vi "Teleop.vi"(10 "Match Info":T3={"Autonomous Elapsed Seconds"=0.0, "TeleOp Elapsed Seconds"=0.0, "Disabled Elapsed Seconds"=0.0, "Visited Autonomous"=FALSE, "Visited TeleOp"=FALSE, "Visited Disabled"=FALSE, "Autonomous Settings"={"Autonomous Style"=enum."Independent", "VI Refnum"=refnum}}, 11 "Call Context":T4) -> ()   [LabVIEW 2020]
doc: "This VI is called for each TeleOp packet received from the DS where the robot is not disabled. It is often used to read from the joysticks and update I/O or to update setpoints for timed control loops. It should complete and return within 20 milliseconds or it may miss DS packets."
uses:
  <vilib>/Rock Robotics/WPI/DriverStation/WPI_DriverStationDerivedRobotMode.ctl
  <vilib>/Rock Robotics/WPI/DriverStation/WPI_DriverStationMatch Info.ctl
  <vilib>/Rock Robotics/WPI/Solenoid/WPI_SolenoidValue.ctl
  <vilib>/Rock Robotics/WPI/ThirdParty/Phoenix-LabVIEW/Motor Controller/Controls/CTRE_Phoenix_MotorControl_ControlMode.ctl
  <vilib>/Rock Robotics/WPI/Utilities/WPI_GetSetVariantRefNum.vi
  <vilib>/Rock Robotics/WPI/ThirdParty/Phoenix-LabVIEW/Pigeon IMU/CTRE_PigeonIMU_GetYPR.vi
  <vilib>/Rock Robotics/Network Tables/NT Read Boolean.vi
  <vilib>/Rock Robotics/Network Tables/NT Read Number.vi
  <vilib>/Rock Robotics/Network Tables/NT Write String.vi
  <vilib>/Rock Robotics/Network Tables/NT Read String.vi
  <vilib>/Rock Robotics/Network Tables/NT Write Boolean.vi
  <vilib>/Rock Robotics/WPI/Solenoid/WPI_SolenoidSetEnum.vi
  <vilib>/Rock Robotics/WPI/ThirdParty/Phoenix-LabVIEW/Motor Controller/Get/CTRE_Phoenix_MotorController_IntegratedSensorData_TalonFX.vi
  <vilib>/Rock Robotics/WPI/ThirdParty/Phoenix-LabVIEW/CANCoder/Get/CTRE_Phoenix_CANcoder_GetSensorData.vi
  <vilib>/addons/control/pid/pid.llb/PID (DBL).vi
  <vilib>/addons/control/pid/NI_PID_pid.lvlib
panel:
  in  "ballCount":dbl
  out "Pigeon Value":dbl
  out "frontrightmotor":dbl
  out "frontleftdrive":dbl
  in  "PID gains 4":T1={"proportional gain (Kc)"=-0.01, "integral time (Ti, min)"=0.0, "derivative time (Td, min)"=2e-05} {"derivative time (Td, min)" format="%.6f"; "integral time (Ti, min)" format="%.6f"; "proportional gain (Kc)" format="%.6f"}
  in  "PID gains 3":T1={"proportional gain (Kc)"=0.01, "integral time (Ti, min)"=0.0, "derivative time (Td, min)"=2e-05} {"derivative time (Td, min)" format="%.6f"; "integral time (Ti, min)" format="%.6f"; "proportional gain (Kc)" format="%.6f"}
  in  "PID gains 2":T1={"proportional gain (Kc)"=-0.01, "integral time (Ti, min)"=0.0, "derivative time (Td, min)"=2e-05} {"derivative time (Td, min)" format="%.6f"; "integral time (Ti, min)" format="%.6f"; "proportional gain (Kc)" format="%.6f"}
  in  "PID gains":T1={"proportional gain (Kc)"=0.01, "integral time (Ti, min)"=0.0, "derivative time (Td, min)"=2e-05} {"derivative time (Td, min)" format="%.6f"; "integral time (Ti, min)" format="%.6f"; "proportional gain (Kc)" format="%.6f"}
  out "Motor out 4":dbl
  out "Desired Position 4":dbl
  out "Motor out 1":dbl
  out "Desired Position 1":dbl
  out "Motor Out 2":dbl
  out "Desired Position 2":dbl
  out "Motor out 3":dbl
  out "Desired Position 3":dbl
  out "Sensor Position 4":dbl
  out "Sensor Position 3":dbl
  out "Sensor Position 2":dbl
  out "Sensor Position 1":dbl
  out "Rotation steering angle 4":dbl
  out "WheelDirection4":dbl(knob) scale=180.0..-180.0
  out "Throttle 4":dbl(slide) scale=-1.0..1.0
  out "Y4":dbl
  out "X4":dbl
  out "Rotation steering angle 3":dbl
  out "WheelDirection3":dbl(knob) scale=180.0..-180.0
  out "Throttle 3":dbl(slide) scale=-1.0..1.0
  out "Y3":dbl
  out "X3":dbl
  out "Rotation steering angle 2":dbl
  out "WheelDirection2":dbl(knob) scale=180.0..-180.0
  out "Throttle 2":dbl(slide) scale=-1.0..1.0
  out "Y2":dbl
  out "X2":dbl
  out "Rotation steering angle 1":dbl
  out "WheelDirection1":dbl(knob) scale=180.0..-180.0
  out "Throttle 1":dbl(slide) scale=-1.0..1.0
  out "Y1":dbl
  out "X1":dbl
  out "Z - Axis":dbl
  out "Y - Axis":dbl
  out "X - Axis":dbl
  in  "Turret 2":dbl format="%#_13g"
  in  "Turret 1":dbl
  in  "Shoot %":dbl
  out "Limit 2":bool
  out "Limit 1":bool
  in  "intake press":T2=enum."Forward"
  in  "intake not press":T2=enum."Reverse"
  out "Position":dbl format="%.2f"
  in  "Elevate Wanted":dbl
  out "Elevate Pressed":bool
  out "Reject Pressed Count":i32
  in  "Elevate (not wanted)":dbl format="%#_13g"
  in  "Intake (wanted)":dbl=1.0 format="%#_13g"
  in  "Reject (wanted)":dbl=-1.0 format="%#_13g"
  in  "Reject (not wanted)":dbl
  in  "Intake (not wanted)":dbl
  in  "Auto-Accept":bool
  in  "8togglePressed?":bool
  in  "Red/Blue":u32(colorbox)
  out "B":u8
  out "G":u8
  out "R":u8
  out "Color":u32(colorbox)
  out "Sample Slider 0":dbl(slide) scale=0.0..5.0
  out "Sample Boolean 1":bool
  out "Sample Boolean 0":bool
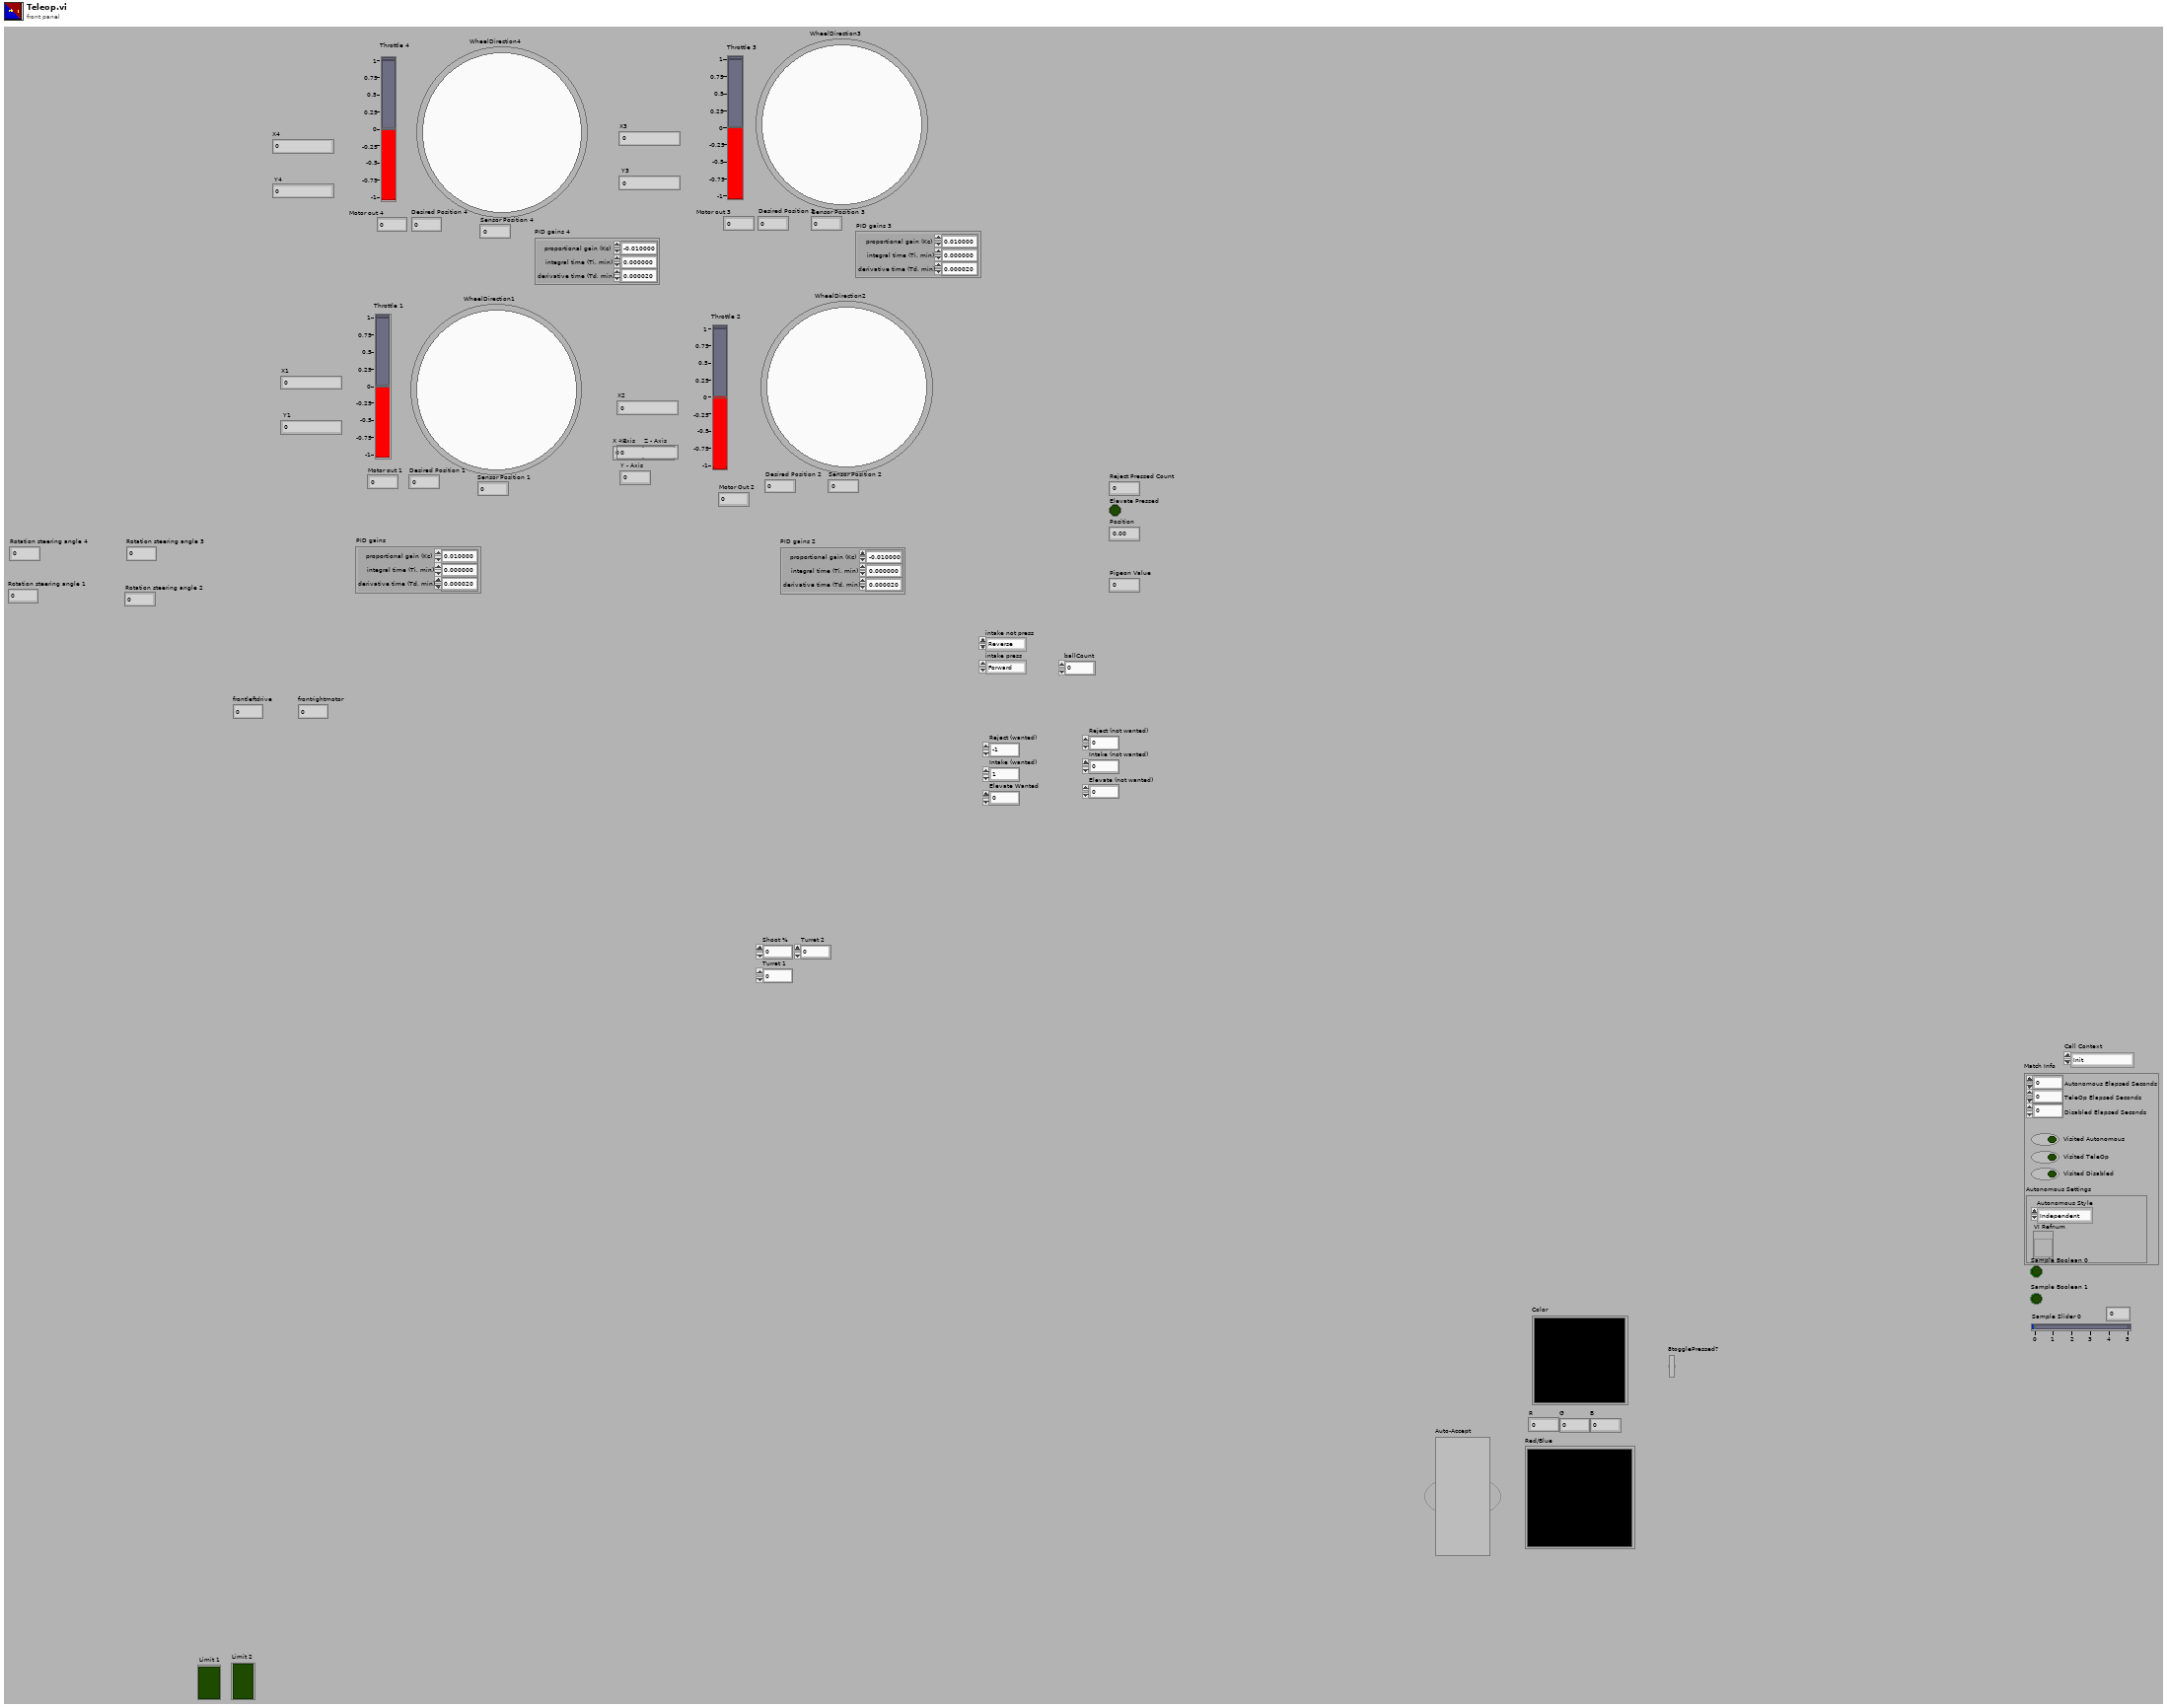
[diagram p1: front panel]
types:
  T1 = cluster{"proportional gain (Kc)":dbl, "integral time (Ti, min)":dbl, "derivative time (Td, min)":dbl}
  T2 = typedef "WPI_SolenoidValue.ctl" = enum16{"Off", "On", "Forward", "Reverse"}
  T3 = typedef "WPI_DriverStationMatch Info.ctl" = cluster{"Autonomous Elapsed Seconds":dbl, "TeleOp Elapsed Seconds":dbl, "Disabled Elapsed Seconds":dbl, "Visited Autonomous":bool, "Visited TeleOp":bool, "Visited Disabled":bool, "Autonomous Settings":cluster{"Autonomous Style":enum16{"Iterative", "Independent"}, "VI Refnum":refnum<vi>}}
  T4 = typedef "WPI_DriverStationDerivedRobotMode.ctl" = enum16{"Init", "Execute", "Stop"}
  T5 = typedef "CTRE_Phoenix_MotorControl_ControlMode.ctl" = u16
  T6 = typedef "WPI_MotorControlDeviceRef.ctl" = cluster{"DeviceStatus":errorcluster, "Type":T7, "PWM":cluster{"PWM Channel":T8, "DeadBand":T9}, "CAN":cluster{"Device Number":u8, "SetOutput VI Ref":variant, "GetOutput VI Ref":variant, "Enable VI Ref":variant, "Disable VI Ref":variant, "Data":variant}, "Invert":bool, "DIO PWM":cluster{"PWM \"Enable\" Channel":T8, "DIOChannel":T10, "PWM Rate":dbl}}
  T7 = typedef "WPI_MotorControlType.ctl" = enum16{"PWM", "CAN", "DIO PWM"}
  T8 = typedef "FPGA_DIOPWMChannel.ctl" = enum8{"PWM 0", "PWM 1", "PWM 2", "PWM 3", "PWM 4", "PWM 5", "PWM 6", "PWM 7", "PWM 8", "PWM 9", "PWM MXP 0", "PWM MXP 1", "PWM MXP 2", "PWM MXP 3", "PWM MXP 4", "PWM MXP 5", "PWM MXP 6", "PWM MXP 7", "PWM MXP 8", "PWM MXP 9", "Invalid"}
  T9 = typedef "WPI_PWMDeadband.ctl" = cluster{"Name":string, "maxPositivePwm":i32, "minPositivePwm":i32, "centerPwm":i32, "maxNegativePwm":i32, "minNegativePwm":i32, "angularRange":u16}
  T10 = typedef "FPGA_DIOChannel.ctl" = enum8{"DIO 0", "DIO 1", "DIO 2", "DIO 3", "DIO 4", "DIO 5", "DIO 6", "DIO 7", "DIO 8", "DIO 9", "DIO MXP 0", "DIO MXP 1", "DIO MXP 2", "DIO MXP 3", "DIO MXP 4", "DIO MXP 5", "DIO MXP 6", "DIO MXP 7", "DIO MXP 8", "DIO MXP 9", "DIO MXP 10", "DIO MXP 11", "DIO MXP 12", "DIO MXP 13", "DIO MXP 14", "DIO MXP 15", "SPI Port CS1", "SPI Port CS2", "SPI Port CS3", "SPI Port MISO", "SPI Port MOSI", "Invalid"}
  T11 = typedef "WPI_SwitchDevRef.ctl" = cluster{"DevStatus":errorcluster, "DIO Channel":T10, "CntIndex":T12, "Normally Closed":bool}
  T12 = typedef "FPGA_CounterCtrSystemIndex.ctl" = enum8{"Ctr 0", "Ctr 1", "Ctr 2", "Ctr 3", "Ctr 4", "Ctr 5", "Ctr 6", "Ctr 7", "Invalid"}
  T13 = typedef "WPI_SolenoidDevRef.ctl" = cluster{"DevStatus":errorcluster, "Pneumatics Control Module":u8, "Forward Solenoid Channel":T14, "Reverse Solenoid Channel":T14}
  T14 = typedef "WPI_SolenoidChannel.ctl" = enum8{"Solenoid 0", "Solenoid 1", "Solenoid 2", "Solenoid 3", "Solenoid 4", "Solenoid 5", "Solenoid 6", "Solenoid 7", "Solenoid 8", "Solenoid 9", "Solenoid 10", "Solenoid 11", "Solenoid 12", "Solenoid 13", "Solenoid 14", "Solenoid 15", "Invalid"}
  T15 = typedef "Color Sensor V3 DevRef.ctl" = cluster{"I2CDevRef":T16}
  T16 = typedef "WPI_I2CDevRef.ctl" = cluster{"DevStatus":errorcluster, "Device Address":u8, "Handle":i32, "I2C Bus":T17}
  T17 = typedef "i2c_bus.ctl" = enum16{"I2C On-Board", "I2C MXP", "Invalid"}
  T18 = typedef "WPI_JoystickDevRef.ctl" = cluster{"Device":T19}
  T19 = typedef "WPI_JoystickDeviceEnum.ctl" = enum16{"USB 0", "USB 1", "USB 2", "USB 3", "USB 4", "USB 5"}
  T20 = typedef "CTRE_PigeonIMU_DeviceRef.ctl" = cluster{"DeviceStatus":errorcluster, "Device Number":u8, "Type":T21, "Device ID":u32, "Handle":u64, "UsageFrame":u32, "Library Path":path}
  T21 = typedef "CTRE_PigeonIMU_ConnectionType.ctl" = u32
  T22 = typedef "WPI_CompressorDevRef.ctl" = cluster{"DevStatus":errorcluster, "Pneumatics Control Module":u8}
  T23 = typedef "CTRE_Phoenix_CANcoder_DeviceRef.ctl" = cluster{"DeviceStatus":errorcluster, "Device Number":u8, "Handle":u64, "UsageFrame":u32, "Library Path":path}
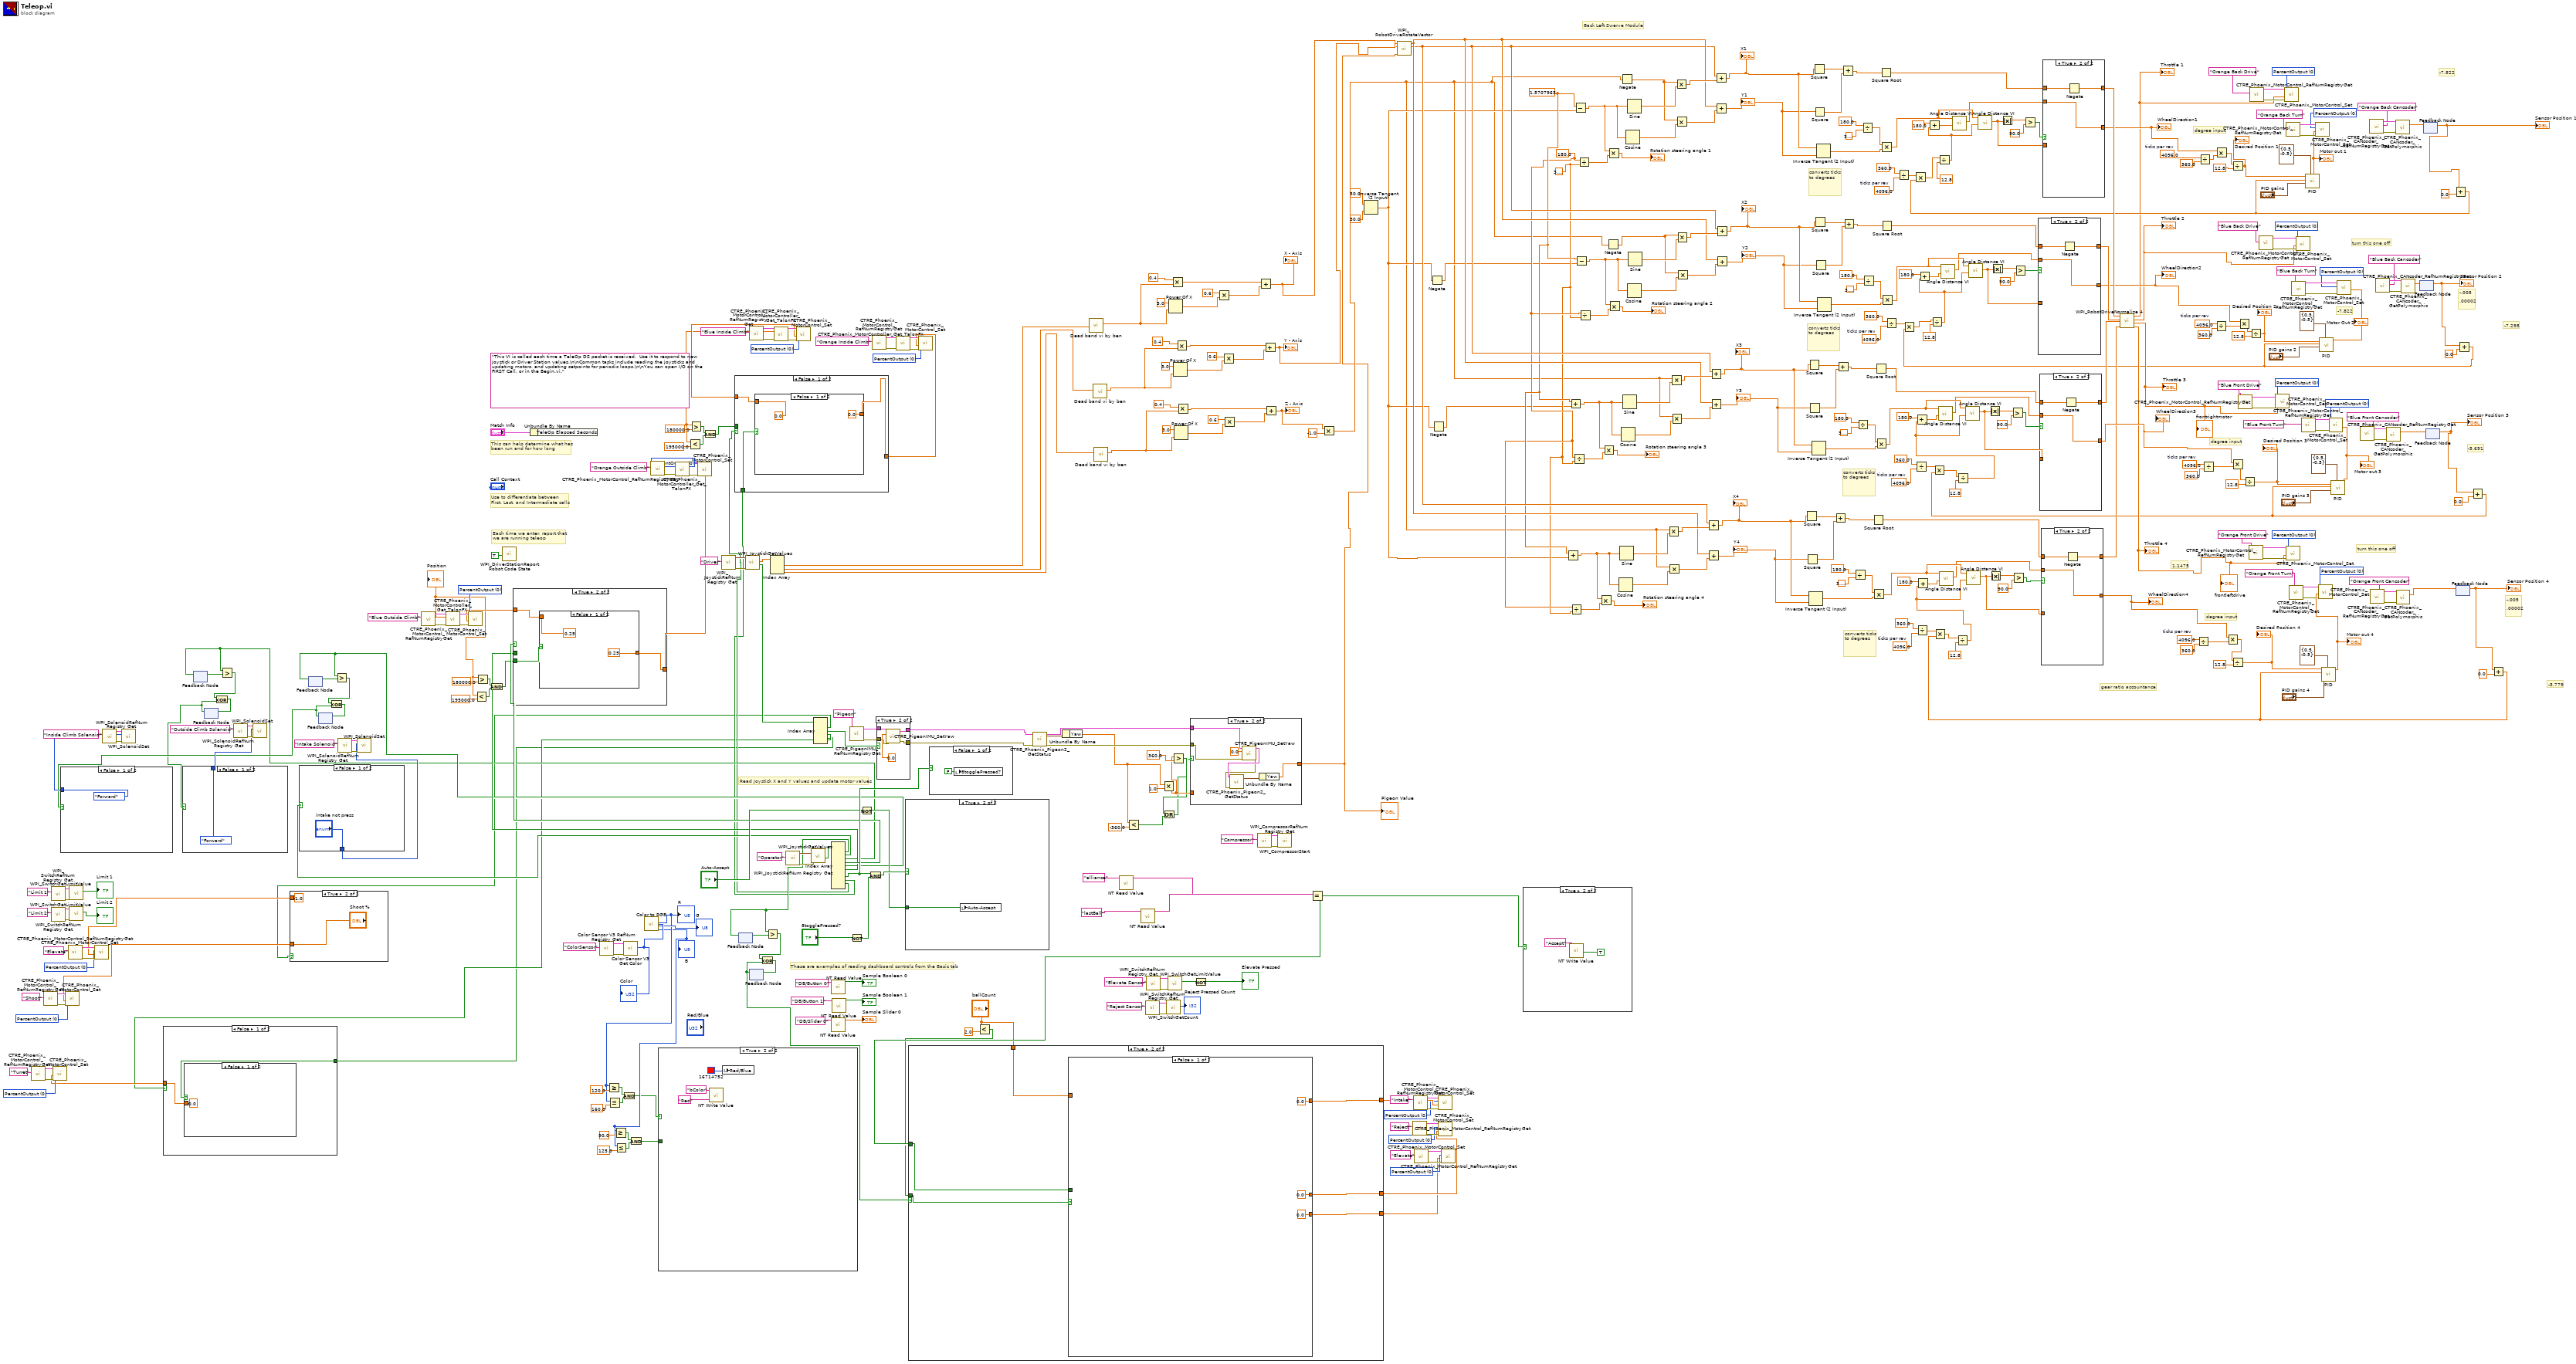
[diagram p0: block diagram]
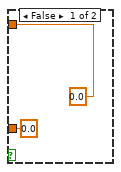
[diagram p2: hidden frame]
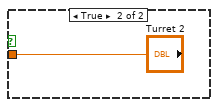
[diagram p8: hidden frame]
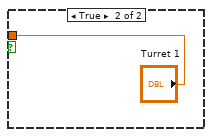
[diagram p9: hidden frame]
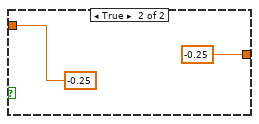
[diagram p10: hidden frame]
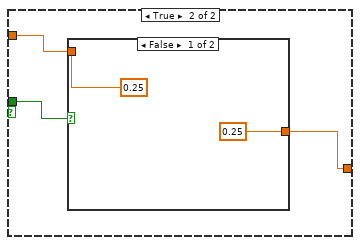
[diagram p11: hidden frame]
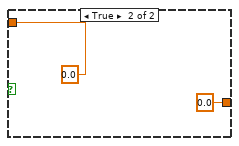
[diagram p12: hidden frame]
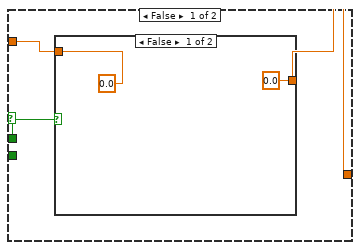
[diagram p13: hidden frame]
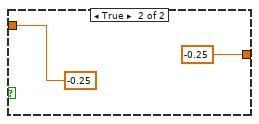
[diagram p14: hidden frame]
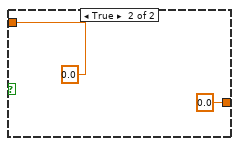
[diagram p15: hidden frame]
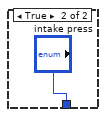
[diagram p16: hidden frame]
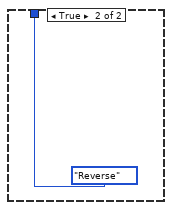
[diagram p17: hidden frame]
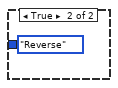
[diagram p18: hidden frame]
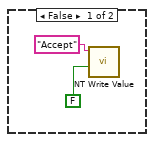
[diagram p19: hidden frame]
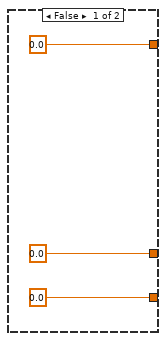
[diagram p20: hidden frame]
diagram:
  w20 = T5 0 items=["PercentOutput"=0, "Position"=1, "Velocity"=2, "Current"=3, "Follower"=5, "MotionProfile"=6, "MotionMagic"=7, "MotionProfileArc"=10, "Disabled"=15] ("Control Mode")
  w102 = T5 0 items=["PercentOutput"=0, "Position"=1, "Velocity"=2, "Current"=3, "Follower"=5, "MotionProfile"=6, "MotionMagic"=7, "MotionProfileArc"=10, "Disabled"=15] ("Control Mode")
  w114 = T5 0 items=["PercentOutput"=0, "Position"=1, "Velocity"=2, "Current"=3, "Follower"=5, "MotionProfile"=6, "MotionMagic"=7, "MotionProfileArc"=10, "Disabled"=15] ("Control Mode")
  w115 = T5 0 items=["PercentOutput"=0, "Position"=1, "Velocity"=2, "Current"=3, "Follower"=5, "MotionProfile"=6, "MotionMagic"=7, "MotionProfileArc"=10, "Disabled"=15] ("Control Mode")
  w116 = T5 0 items=["PercentOutput"=0, "Position"=1, "Velocity"=2, "Current"=3, "Follower"=5, "MotionProfile"=6, "MotionMagic"=7, "MotionProfileArc"=10, "Disabled"=15] ("Control Mode")
  w117 = T5 0 items=["PercentOutput"=0, "Position"=1, "Velocity"=2, "Current"=3, "Follower"=5, "MotionProfile"=6, "MotionMagic"=7, "MotionProfileArc"=10, "Disabled"=15] ("Control Mode")
  w118 = T5 0 items=["PercentOutput"=0, "Position"=1, "Velocity"=2, "Current"=3, "Follower"=5, "MotionProfile"=6, "MotionMagic"=7, "MotionProfileArc"=10, "Disabled"=15] ("Control Mode")
  w119 = T5 0 items=["PercentOutput"=0, "Position"=1, "Velocity"=2, "Current"=3, "Follower"=5, "MotionProfile"=6, "MotionMagic"=7, "MotionProfileArc"=10, "Disabled"=15] ("Control Mode")
  w120 = T5 0 items=["PercentOutput"=0, "Position"=1, "Velocity"=2, "Current"=3, "Follower"=5, "MotionProfile"=6, "MotionMagic"=7, "MotionProfileArc"=10, "Disabled"=15] ("Control Mode")
  w132 = 4096.0  # ticks per rev
  w145 = 4096.0  # ticks per rev
  w159 = 4096.0  # ticks per rev
  w170 = 4096.0  # ticks per rev
  w62 = 1.5707963 ("y")
  w181 = 4096.0  # ticks per rev
  w185 = 4096.0  # ticks per rev
  w189 = 4096.0  # ticks per rev
  w105 = 4096.0  # ticks per rev
  w60 = 3.141592653589793
  w61 = 180.0 ("x")
  w299 = T5 0 items=["PercentOutput"=0, "Position"=1, "Velocity"=2, "Current"=3, "Follower"=5, "MotionProfile"=6, "MotionMagic"=7, "MotionProfileArc"=10, "Disabled"=15] ("Control Mode")
  w303 = T5 0 items=["PercentOutput"=0, "Position"=1, "Velocity"=2, "Current"=3, "Follower"=5, "MotionProfile"=6, "MotionMagic"=7, "MotionProfileArc"=10, "Disabled"=15] ("Control Mode")
  w327 = T5 0 items=["PercentOutput"=0, "Position"=1, "Velocity"=2, "Current"=3, "Follower"=5, "MotionProfile"=6, "MotionMagic"=7, "MotionProfileArc"=10, "Disabled"=15] ("Control Mode")
  w328 = T5 0 items=["PercentOutput"=0, "Position"=1, "Velocity"=2, "Current"=3, "Follower"=5, "MotionProfile"=6, "MotionMagic"=7, "MotionProfileArc"=10, "Disabled"=15] ("Control Mode")
  w329 = T5 0 items=["PercentOutput"=0, "Position"=1, "Velocity"=2, "Current"=3, "Follower"=5, "MotionProfile"=6, "MotionMagic"=7, "MotionProfileArc"=10, "Disabled"=15] ("Control Mode")
  w369 = T5 0 items=["PercentOutput"=0, "Position"=1, "Velocity"=2, "Current"=3, "Follower"=5, "MotionProfile"=6, "MotionMagic"=7, "MotionProfileArc"=10, "Disabled"=15] ("Control Mode")
  w402 = T5 0 items=["PercentOutput"=0, "Position"=1, "Velocity"=2, "Current"=3, "Follower"=5, "MotionProfile"=6, "MotionMagic"=7, "MotionProfileArc"=10, "Disabled"=15] ("Control Mode")
  w403 = T5 0 items=["PercentOutput"=0, "Position"=1, "Velocity"=2, "Current"=3, "Follower"=5, "MotionProfile"=6, "MotionMagic"=7, "MotionProfileArc"=10, "Disabled"=15] ("Control Mode")
  w407 = T5 0 items=["PercentOutput"=0, "Position"=1, "Velocity"=2, "Current"=3, "Follower"=5, "MotionProfile"=6, "MotionMagic"=7, "MotionProfileArc"=10, "Disabled"=15] ("Control Mode")
  (unwired) "This VI is called each time a TeleOp DS packet is received.  Use it to respond to new joystick or Driver Station values.\n\nCommon tasks include reading the joysticks and updating motors, and updating setpoints for periodic loops.\n\nYou can open I/O on the FIRST Call, or in the Begin.vi."
  # "-.005\n\n.00002"
  # "-.005\n\n.00002"
  # "-7.822"
  # "-7.295"
  # "-3.691"
  # "-3.779"
  # "1.1475"
  # "turn this one off"
  # "turn this one off"
  # "gear ratio accountance"
  # "converts ticks to degrees"
  # "converts ticks to degrees"
  # "converts ticks to degrees"
  # "converts ticks to degrees"
  # "degree input"
  # "degree input"
  # "degree input"
  # "Back Left Swerve Module"
  # "These are examples of reading dashboard controls from the Basic tab"
  # "Read Joystick X and Y values and update motor values"
  # "-7.822"
  # "Each time we enter, report that\nwe are running teleop"
  # "Use to differentiate between\nFirst, Last, and Intermediate calls"
  # "This can help determine what has\nbeen run and for how long"
  n1 = call <vilib>:"CTRE_Phoenix_MotorControl_RefNumRegistryGet.vi"("refnum name"="Turret") -> ("error out"=w302:errorcluster, "PhoenixMotorControlDevRef"=w301:T6)  [unwired: 9 in]
  n2 = call <vilib>:"CTRE_Phoenix_MotorControl_RefNumRegistryGet.vi"("refnum name"="Shoot") -> ("error out"=w306:errorcluster, "PhoenixMotorControlDevRef"=w305:T6)  [unwired: 9 in]
  n3 = call <vilib>:"WPI_SwitchRefNum Registry Get.vi"("refnum name"="Limit 1") -> ("error out"=w314:errorcluster, "SwitchDevRef"=w313:T11)  [unwired: 9 in]
  n4 = call <vilib>:"WPI_SwitchRefNum Registry Get.vi"("refnum name"="Limit 2") -> ("error out"=w311:errorcluster, "SwitchDevRef"=w310:T11)  [unwired: 9 in]
  n5 = call <vilib>:"CTRE_Phoenix_MotorControl_RefNumRegistryGet.vi"("refnum name"="Elevate") -> ("error out"=w22:errorcluster, "PhoenixMotorControlDevRef"=w19:T6)  [unwired: 9 in]
  n6 = call <vilib>:"WPI_SwitchGetLimitValue.vi"("error in (no error)"=w314, "SwitchDevRef"=w313) -> ("Switch Pressed"=→"Limit 1":bool)  [unwired: 7 in, 2 out]
  n7 = call <vilib>:"WPI_SwitchGetLimitValue.vi"("error in (no error)"=w311, "SwitchDevRef"=w310) -> ("Switch Pressed"=→"Limit 2":bool)  [unwired: 7 in, 2 out]
  n8 = call <vilib>:"WPI_SolenoidRefNum Registry Get.vi"("refnum name"="Inside Climb Solenoid") -> ("error out"=w386:errorcluster, "SolenoidDevRef"=w385:T13)  [unwired: 9 in]
  n9 = feedback #1() -> (w349:bool)  [unwired: 1 in]
  n10 = feedback #2() -> (w345:bool)  [unwired: 1 in]
  n11 = case shown="False" w345 {
    tunnel: [WPI_SolenoidValue."Forward" ("Value") WPI_SolenoidValue."Reverse" ("Value")] -> w376
    frame False {
    }
    frame True {
    }
  }
  n12 = call <vilib>:"WPI_SolenoidRefNum Registry Get.vi"("refnum name"="Outside Climb Solenoid") -> ("error out"=w384:errorcluster, "SolenoidDevRef"=w383:T13)  [unwired: 9 in]
  n13 = call-poly <vilib>:"WPI_SolenoidSet.vi"("error in (no error)"=w384, "Value"=w376, "SolenoidDevRef"=w383) -> ()  [unwired: 7 in, 2 out]
  n14 = feedback #3() -> (w354:bool)  [unwired: 1 in]
  n15 = feedback #4() -> (w350:bool)  [unwired: 1 in]
  n16 = case shown="False" w350 {
    tunnel: [WPI_SolenoidValue."Forward" ("Value") WPI_SolenoidValue."Reverse" ("Value")] -> w377
    frame False {
    }
    frame True {
    }
  }
  n17 = call-poly <vilib>:"WPI_SolenoidSet.vi"("error in (no error)"=w386, "Value"=w377, "SolenoidDevRef"=w385) -> ()  [unwired: 7 in, 2 out]
  n18 = call <vilib>:"WPI_SolenoidRefNum Registry Get.vi"("refnum name"="Intake Solenoid") -> ("error out"=w382:errorcluster, "SolenoidDevRef"=w381:T13)  [unwired: 9 in]
  n19 = call <vilib>:"CTRE_Phoenix_MotorControl_RefNumRegistryGet.vi"("refnum name"="Blue Outside Climb") -> ("error out"=w372:errorcluster, "PhoenixMotorControlDevRef"=w373:T6)  [unwired: 9 in]
  n20 = call-poly <vilib>:"CTRE_Phoenix_MotorController_Get_TalonFX.vi"("PhoenixMotorControlDevRef"=w373, "error in"=w372) -> ("PhoenixMotorControlDevRef"=w370:T6, "Position"=w362:dbl, "error out"=w371:errorcluster)  [unwired: 9 in, 2 out]
  "Position" <- w362
  n21 = Less?(x=w362, y=195000.0) -> (x < y?=w363:bool)
  n22 = Greater?(x=w362, y=180000.0) -> (0:w364:bool)
  n23 = And(x=w364, y=w363) -> (x .and. y?=w317:bool)
  n24 = call <vilib>:"WPI_DriverStationReport Robot Code State.vi"("TeleOp"=TRUE ("Autonomous")) -> ()  [unwired: 10 in, 1 out]
  n25 = Unbundle By Name("Match Info") -> ()  [unwired: 1 out]
  n26 = call <vilib>:"Color Sensor V3 RefNum Registry Get.vi"("refnum name"="ColorSensor") -> ("error out"=w441:errorcluster, "ColorSensorDevRef"=w442:T15)  [unwired: 9 in]
  n27 = call <vilib>:"Color Sensor V3 Get Color.vi"("error in (no error)"=w441, "ColorSensorDevRef"=w442) -> ("Color"=w440:u32)  [unwired: 6 in, 3 out]
  "Color" <- w440
  n28 = call <vilib>:"Color to RGB.vi"("Color"=w440) -> ("R"=w434:u8, "G"=→"G":u8, "B"=w429:u8)  [unwired: 1 out]
  "R" <- w434
  "B" <- w429
  n29 = Greater Or Equal?(x=w434, y=120.0) -> (x >= y?=w437:bool)
  n30 = Less Or Equal?(x=w434, y=160.0) -> (x <= y?=w438:bool)
  n31 = Greater Or Equal?(x=w429, y=90.0) -> (x >= y?=w432:bool)
  n32 = Less Or Equal?(x=w429, y=125.0) -> (x <= y?=w433:bool)
  n33 = And(x=w437, y=w438) -> (x .and. y?=w418:bool)
  n34 = And(x=w432, y=w433) -> (x .and. y?=w417:bool)
  n35 = call <vilib>:"CTRE_Phoenix_MotorControl_RefNumRegistryGet.vi"("refnum name"="Orange Outside Climb") -> ("error out"=w333:errorcluster, "PhoenixMotorControlDevRef"=w334:T6)  [unwired: 9 in]
  n36 = case shown="True" w418 {
    tunnel: w417 -> [w469 _]
    frame False {
      n37 = case shown="True" w469 {
        frame False {
          n38 = call-poly <vilib>:"NT Write Value.vi"("String"="Empty", "Name"="bColor") -> ()  [unwired: 9 in, 1 out]
          n39 = local write "Red/Blue"(u32 328965 ("Color Box")) -> ()
        }
        frame True {
          n40 = local write "Red/Blue"(u32 1507583 ("Color Box")) -> ()
          n41 = call-poly <vilib>:"NT Write Value.vi"("String"="Blue", "Name"="bColor") -> ()  [unwired: 9 in, 1 out]
        }
      }
    }
    frame True {
      n42 = call-poly <vilib>:"NT Write Value.vi"("String"="Red", "Name"="bColor") -> ()  [unwired: 9 in, 1 out]
      n43 = local write "Red/Blue"(u32 16714752) -> ()
    }
  }
  n44 = call-poly <vilib>:"CTRE_Phoenix_MotorController_Get_TalonFX.vi"("PhoenixMotorControlDevRef"=w334, "error in"=w333) -> ("PhoenixMotorControlDevRef"=w331:T6, "error out"=w332:errorcluster)  [unwired: 9 in, 3 out]
  n45 = call <vilib>:"WPI_JoystickRefNum Registry Get.vi"("refnum name"="Driver") -> ("error out"=w462:errorcluster, "JoystickDevRef"=w461:T18)  [unwired: 9 in]
  n46 = feedback #5() -> (w359:bool)  [unwired: 1 in]
  n47 = call <vilib>:"WPI_JoystickGetValues.vi"("error in (no error)"=w462, "JoystickDevRef"=w461) -> ("Buttons"=w458:bool[], "Axes"=w459:dbl[])  [unwired: 5 in, 3 out]
  n48 = call <vilib>:"CTRE_Phoenix_MotorControl_RefNumRegistryGet.vi"("refnum name"="Blue Inside Climb") -> ("error out"=w338:errorcluster, "PhoenixMotorControlDevRef"=w339:T6)  [unwired: 9 in]
  n49 = feedback #6() -> (w355:bool)  [unwired: 1 in]
  n50 = Index Array(array=w459) -> (element #1=w25:dbl, element #2=w24:dbl, element #3=w23:dbl)  [unwired: 3 in]
  n51 = call-poly <vilib>:"CTRE_Phoenix_MotorController_Get_TalonFX.vi"("PhoenixMotorControlDevRef"=w339, "error in"=w338) -> ("PhoenixMotorControlDevRef"=w336:T6, "Position"=w318:dbl, "error out"=w337:errorcluster)  [unwired: 9 in, 2 out]
  n52 = Less?(x=w318, y=195000.0) -> (x < y?=w321:bool)
  n53 = Greater?(x=w318, y=180000.0) -> (0:w322:bool)
  n54 = And(x=w322, y=w321) -> (x .and. y?=w316:bool)
  n55 = call <vilib>:"WPI_JoystickRefNum Registry Get.vi"("refnum name"="Operator") -> ("error out"=w427:errorcluster, "JoystickDevRef"=w426:T18)  [unwired: 9 in]
  n56 = call <vilib>:"WPI_JoystickGetValues.vi"("error in (no error)"=w427, "JoystickDevRef"=w426) -> ("Buttons"=w425:bool[])  [unwired: 5 in, 4 out]
  n57 = Index Array(array=w458) -> (element #1=w4:bool, element #2=w455:bool, element #3=w297:bool, element #4=w296:bool)  [unwired: 5 in, 1 out]
  n58 = case shown="False" w297 {
    tunnel: [w480 "Turret 1"] -> w298
    tunnel: w296 -> [w479 _]
    frame False {
      n59 = case shown="False" w479 {
        tunnel: [0.0 ("Turret 2") "Turret 2"] -> w480
        frame False {
        }
        frame True {
        }
      }
    }
    frame True {
    }
  }
  n60 = call <vilib>:"CTRE_Phoenix_MotorControl_Set.vi"("error in (no error)"=w302, "Output"=w298, "Control Mode"=w299, "PhoenixMotorControlDevRef"=w301) -> ()  [unwired: 6 in, 2 out]
  n61 = case shown="True" w4 {
    tunnel: [0.0 ("Shoot %") "Shoot %"] -> w6
    tunnel: [0.0 ("Output") -1.0 ("Output")] -> w5
    frame False {
    }
    frame True {
    }
  }
  n62 = call <vilib>:"CTRE_Phoenix_MotorControl_Set.vi"("error in (no error)"=w306, "Output"=w6, "Control Mode"=w303, "PhoenixMotorControlDevRef"=w305) -> ()  [unwired: 6 in, 2 out]
  n63 = call <vilib>:"CTRE_Phoenix_MotorControl_Set.vi"("error in (no error)"=w22, "Output"=w5, "Control Mode"=w20, "PhoenixMotorControlDevRef"=w19) -> ()  [unwired: 6 in, 2 out]
  n64 = Index Array(array=w425) -> (element #1=w358:bool, element #2=w374:bool, element #3=w346:bool, element #4=w367:bool, element #5=w351:bool, element #6=w365:bool, element #8=w420:bool, element #9=w315:bool, element #10=w325:bool)  [unwired: 11 in, 2 out]
  n65 = feedback-in #1(w346) -> ()
  n66 = Greater?(x=w346, y=w349) -> (0:w348:bool)
  n67 = Exclusive Or(1:w345, 2:w348) -> (0:w347:bool)
  n68 = feedback-in #2(w347) -> ()
  n69 = case shown="False" w374 {
    tunnel: ["intake not press" "intake press"] -> w375
    frame False {
    }
    frame True {
    }
  }
  n70 = feedback-in #3(w351) -> ()
  n71 = Greater?(x=w351, y=w354) -> (0:w353:bool)
  n72 = Exclusive Or(1:w350, 2:w353) -> (0:w352:bool)
  n73 = feedback-in #4(w352) -> ()
  n74 = call-poly <vilib>:"WPI_SolenoidSet.vi"("error in (no error)"=w382, "Value"=w375, "SolenoidDevRef"=w381) -> ()  [unwired: 7 in, 2 out]
  n75 = case shown="True" w367 {
    tunnel: [w492 w498] -> w366
    tunnel: w317 -> [_ w499]
    tunnel: w365 -> [w491 _]
    tunnel: [w490 w497] -> w326
    frame False {
      n76 = case shown="False" w491 {
        tunnel: [0.0 ("Output") -0.25 ("Output")] -> w492
        tunnel: [0.0 ("Output") -0.25 ("Output")] -> w490
        frame False {
        }
        frame True {
        }
      }
    }
    frame True {
      n77 = case shown="False" w499 {
        tunnel: [0.25 ("Output") 0.0 ("Output")] -> w498
        tunnel: [0.25 ("Output") 0.0 ("Output")] -> w497
        frame False {
        }
        frame True {
        }
      }
    }
  }
  n78 = call <vilib>:"CTRE_Phoenix_MotorControl_Set.vi"("error in (no error)"=w371, "Output"=w366, "Control Mode"=w369, "PhoenixMotorControlDevRef"=w370) -> ()  [unwired: 6 in, 2 out]
  n79 = call <vilib>:"CTRE_Phoenix_MotorControl_Set.vi"("error in (no error)"=w332, "Output"=w326, "Control Mode"=w327, "PhoenixMotorControlDevRef"=w331) -> ()  [unwired: 6 in, 2 out]
  n80 = case shown="False" w325 {
    tunnel: [w506 w513] -> w324
    tunnel: [w505 w512] -> w323
    tunnel: w315 -> [w504 _]
    tunnel: w316 -> [_ w511]
    frame False {
      n81 = case shown="False" w504 {
        tunnel: [0.0 ("Output") -0.25 ("Output")] -> w506
        tunnel: [0.0 ("Output") -0.25 ("Output")] -> w505
        frame False {
        }
        frame True {
        }
      }
    }
    frame True {
      n82 = case shown="False" w511 {
        tunnel: [0.25 ("Output") 0.0 ("Output")] -> w513
        tunnel: [0.25 ("Output") 0.0 ("Output")] -> w512
        frame False {
        }
        frame True {
        }
      }
    }
  }
  n83 = feedback-in #5(w358) -> ()
  n84 = Greater?(x=w358, y=w359) -> (0:w357:bool)
  n85 = Exclusive Or(1:w355, 2:w357) -> (0:w356:bool)
  n86 = feedback-in #6(w356) -> ()
  n87 = call <vilib>:"CTRE_Phoenix_MotorControl_Set.vi"("error in (no error)"=w337, "Output"=w324, "Control Mode"=w328, "PhoenixMotorControlDevRef"=w336) -> ()  [unwired: 6 in, 2 out]
  n88 = call-poly <vilib>:"NT Read Value.vi"("Name"="DB/Button 0" ("refnum name")) -> ("Boolean"=→"Sample Boolean 0":bool)  [unwired: 9 in, 1 out]
  n89 = call-poly <vilib>:"NT Read Value.vi"("Name"="DB/Slider 0" ("refnum name")) -> ("Numeric"=→"Sample Slider 0":dbl)  [unwired: 9 in, 1 out]
  n90 = call-poly <vilib>:"NT Read Value.vi"("Name"="DB/Button 1" ("refnum name")) -> ("Boolean"=→"Sample Boolean 1":bool)  [unwired: 9 in, 1 out]
  n91 = call <vilib>:"CTRE_PigeonIMU_RefNumRegistryGet.vi"("refnum name"="Pigeon") -> ("error out"=w456:errorcluster, "PigeonIMUDevRef"=w457:T20)  [unwired: 9 in]
  n92 = Not(x="8togglePressed?") -> (.not. x?=w423:bool)
  n93 = Not(x="Auto-Accept") -> (.not. x?=w421:bool)
  n94 = And(x=w420, y=w423) -> (x .and. y?=w422:bool)
  n95 = call <vilib>:"CTRE_Phoenix_MotorControl_RefNumRegistryGet.vi"("refnum name"="Orange Inside Climb") -> ("error out"=w343:errorcluster, "PhoenixMotorControlDevRef"=w344:T6)  [unwired: 9 in]
  n96 = case shown="True" w455 {
    tunnel: w457 -> [w519 w523]
    tunnel: [w519 w522] -> w451
    tunnel: w456 -> [w518 w520]
    tunnel: [w518 w521] -> w450
    frame False {
    }
    frame True {
      n97 = call <vilib>:"CTRE_PigeonIMU_SetYaw.vi"("error in (no error)"=w520, "Value"=0.0, "PigeonIMUDevRef"=w523) -> ("error out"=w521:errorcluster, "PigeonIMUDevRef"=w522:T20)  [unwired: 7 in]
    }
  }
  n98 = call-poly <vilib>:"CTRE_Phoenix_MotorController_Get_TalonFX.vi"("PhoenixMotorControlDevRef"=w344, "error in"=w343) -> ("PhoenixMotorControlDevRef"=w341:T6, "error out"=w342:errorcluster)  [unwired: 9 in, 3 out]
  n99 = case shown="True" w422 {
    tunnel: w421 -> [_ w525]
    frame False {
    }
    frame True {
      n100 = local write "Auto-Accept"(w525) -> ()
    }
  }
  n101 = call <vilib>:"CTRE_Phoenix_MotorControl_Set.vi"("error in (no error)"=w342, "Output"=w323, "Control Mode"=w329, "PhoenixMotorControlDevRef"=w341) -> ()  [unwired: 6 in, 2 out]
  n102 = case shown="False" w420 {
    frame False {
      n103 = local write "8togglePressed?"(FALSE ("togglePressed?")) -> ()
    }
    frame True {
      n104 = local write "8togglePressed?"(TRUE ("togglePressed?")) -> ()
    }
  }
  n105 = Less?(x="ballCount", y=2.0) -> (x < y?=w2:bool)
  n106 = call-poly <vilib>:"CTRE_Phoenix_Pigeon2_GetStatus.vi"("error in (no error)"=w450, "PigeonIMUDevRef"=w451) -> ("error out"=w14:errorcluster, "Yaw Pitch Roll"=w452:cluster{"Yaw":dbl, "Pitch":dbl, "Roll":dbl}, "PigeonIMUDevRef"=w15:T20)  [unwired: 7 in]
  n107 = Unbundle By Name(w452) -> ("Yaw"=w11:dbl)
  n108 = call "Dead band vi by ben.vi"("Numeric"=w25) -> ("Deadbanded Value"=w289:dbl)  [unwired: 10 in]
  n109 = call "Dead band vi by ben.vi"("Numeric"=w24) -> ("Deadbanded Value"=w282:dbl)  [unwired: 10 in]
  n110 = call "Dead band vi by ben.vi"("Numeric"=w23) -> ("Deadbanded Value"=w275:dbl)  [unwired: 10 in]
  n111 = call-poly <vilib>:"NT Read Value.vi"("Name"="alliance") -> ("String"=w397:string)  [unwired: 9 in, 1 out]
  n112 = Less?(x=w11, y=-360.0) -> (x < y?=w12:bool)
  n113 = call-poly <vilib>:"NT Read Value.vi"("Name"="lastBall") -> ("String"=w398:string)  [unwired: 9 in, 1 out]
  n114 = call <vilib>:"WPI_SwitchRefNum Registry Get.vi"("refnum name"="Reject Sensor") -> ("error out"=w391:errorcluster, "SwitchDevRef"=w390:T11)  [unwired: 9 in]
  n115 = call <vilib>:"WPI_SwitchRefNum Registry Get.vi"("refnum name"="Elevate Sensor") -> ("error out"=w394:errorcluster, "SwitchDevRef"=w393:T11)  [unwired: 9 in]
  n116 = Multiply(x=w11, y=1.0) -> (x*y=w16:dbl)
  n117 = call <vilib>:"WPI_SwitchGetCount.vi"("error in (no error)"=w391, "SwitchDevRef"=w390) -> ("Switch Pressed Count"=→"Reject Pressed Count":i32)  [unwired: 7 in, 2 out]
  n118 = call <vilib>:"WPI_SwitchGetLimitValue.vi"("error in (no error)"=w394, "SwitchDevRef"=w393) -> ("Switch Pressed"=w387:bool)  [unwired: 7 in, 2 out]
  n119 = Power Of X(1:w289, 2:3.0 ("y")) -> (0:w293:dbl)
  n120 = Multiply(x=0.4, y=w289) -> (x*y=w290:dbl)
  n121 = Greater?(x=w16, y=360.0) -> (0:w13:bool)
  n122 = Or(x=w13, y=w12) -> (x .or. y?=w9:bool)
  n123 = Power Of X(1:w282, 2:3.0 ("y")) -> (0:w286:dbl)
  n124 = Power Of X(1:w275, 2:3.0 ("y")) -> (0:w279:dbl)
  n125 = Multiply(x=0.4, y=w282) -> (x*y=w283:dbl)
  n126 = Multiply(x=0.4, y=w275) -> (x*y=w276:dbl)
  n127 = case shown="True" w9 {
    tunnel: [w528 w529] -> w17
    tunnel: w16 -> [w528 _]
    tunnel: w15 -> [_ w535]
    tunnel: w14 -> [_ w534]
    frame False {
    }
    frame True {
      n128 = call <vilib>:"CTRE_PigeonIMU_SetYaw.vi"("error in (no error)"=w534, "Value"=0.0, "PigeonIMUDevRef"=w535) -> ("error out"=w530:errorcluster, "PigeonIMUDevRef"=w531:T20)  [unwired: 7 in]
      n129 = call-poly <vilib>:"CTRE_Phoenix_Pigeon2_GetStatus.vi"("error in (no error)"=w530, "PigeonIMUDevRef"=w531) -> ("Yaw Pitch Roll"=w532:cluster{"Yaw":dbl, "Pitch":dbl, "Roll":dbl})  [unwired: 7 in, 2 out]
      n130 = Unbundle By Name(w532) -> ("Yaw"=w529:dbl)
    }
  }
  "Pigeon Value" <- w17
  n131 = Not(x=w387) -> (.not. x?=→"Elevate Pressed":bool)
  n132 = Multiply(x=0.6, y=w293) -> (x*y=w291:dbl)
  n133 = Multiply(x=0.6, y=w286) -> (x*y=w284:dbl)
  n134 = Multiply(x=0.6, y=w279) -> (x*y=w277:dbl)
  n135 = call <vilib>:"WPI_CompressorRefNum Registry Get.vi"("refnum name"="Compressor") -> ("error out"=w401:errorcluster, "CompressorDevRef"=w400:T22)  [unwired: 9 in]
  n136 = Add(x=w290, y=w291) -> (x+y=w38:dbl)
  "X - Axis" <- w38
  n137 = Add(x=w283, y=w284) -> (x+y=w39:dbl)
  "Y - Axis" <- w39
  n138 = Add(x=w276, y=w277) -> (x+y=w36:dbl)
  "Z - Axis" <- w36
  n139 = call <vilib>:"WPI_CompressorStart.vi"("error in (no error)"=w401, "CompressorDevRef"=w400) -> ()  [unwired: 8 in, 2 out]
  n140 = Equal?(x=w397, y=w398) -> (x = y?=w8:bool)
  n141 = case shown="True" w355 {
    tunnel: [0.0 ("Output") w542] -> w406
    tunnel: [0.0 ("Output") w544] -> w405
    tunnel: [0.0 ("Output") w543] -> w404
    tunnel: w8 -> [_ w541]
    tunnel: w2 -> [_ w540]
    tunnel: "ballCount" -> [_ w539]
    frame False {
    }
    frame True {
      n142 = case shown="False" w540 {
        tunnel: [0.0 ("Reject (wanted)") w553] -> w544
        tunnel: [0.0 ("Elevate Wanted") w552] -> w543
        tunnel: [0.0 ("Intake (wanted)") w551] -> w542
        tunnel: w541 -> [_ w550]
        tunnel: w539 -> [_ w548]
        frame False {
        }
        frame True {
          n143 = Increment(x=w548) -> (x+1=w549:dbl)
          n144 = local write "ballCount"(w549) -> ()
          n145 = case shown="True" w550 {
            tunnel: ["Reject (not wanted)" "Reject (wanted)"] -> w553
            tunnel: ["Elevate (not wanted)" "Elevate Wanted"] -> w552
            tunnel: ["Intake (not wanted)" "Intake (wanted)"] -> w551
            frame False {
            }
            frame True {
            }
          }
        }
      }
    }
  }
  n146 = Multiply(x=w36, y=-1.0) -> (x*y=w34:dbl)
  n147 = Inverse Tangent (2 Input)(1:30.0 ("x"), 2:30.0 ("y")) -> (0:w52:dbl)
  n148 = call <vilib>:"WPI_RobotDriveRotateVector.vi"("Angle"=w17, "X"=w38, "Y"=w39) -> ("X'"=w211:dbl, "Y'"=w212:dbl)  [unwired: 7 out]
  n149 = call <vilib>:"CTRE_Phoenix_MotorControl_RefNumRegistryGet.vi"("refnum name"="Reject") -> ("error out"=w414:errorcluster, "PhoenixMotorControlDevRef"=w413:T6)  [unwired: 9 in]
  n150 = call <vilib>:"CTRE_Phoenix_MotorControl_RefNumRegistryGet.vi"("refnum name"="Intake") -> ("error out"=w416:errorcluster, "PhoenixMotorControlDevRef"=w415:T6)  [unwired: 9 in]
  n151 = call <vilib>:"CTRE_Phoenix_MotorControl_RefNumRegistryGet.vi"("refnum name"="Elevate") -> ("error out"=w412:errorcluster, "PhoenixMotorControlDevRef"=w411:T6)  [unwired: 9 in]
  n152 = Negate(x=w52) -> (-x=w53:dbl)
  n153 = Negate(x=w52) -> (-x=w51:dbl)
  n154 = call <vilib>:"CTRE_Phoenix_MotorControl_Set.vi"("error in (no error)"=w414, "Output"=w405, "Control Mode"=w402, "PhoenixMotorControlDevRef"=w413) -> ()  [unwired: 6 in, 2 out]
  n155 = call <vilib>:"CTRE_Phoenix_MotorControl_Set.vi"("error in (no error)"=w416, "Output"=w406, "Control Mode"=w403, "PhoenixMotorControlDevRef"=w415) -> ()  [unwired: 6 in, 2 out]
  n156 = call <vilib>:"CTRE_Phoenix_MotorControl_Set.vi"("error in (no error)"=w412, "Output"=w404, "Control Mode"=w407, "PhoenixMotorControlDevRef"=w411) -> ()  [unwired: 6 in, 2 out]
  n157 = case shown="True" w8 {
    frame False {
      n158 = call-poly <vilib>:"NT Write Value.vi"("Boolean"=FALSE, "Name"="Accept") -> ()  [unwired: 9 in, 1 out]
    }
    frame True {
      n159 = call-poly <vilib>:"NT Write Value.vi"("Boolean"=TRUE, "Name"="Accept") -> ()  [unwired: 9 in, 1 out]
    }
  }
  n160 = Add(x=w62, y=w52) -> (x+y=w220:dbl)
  n161 = Add(x=w62, y=w51) -> (x+y=w235:dbl)
  n162 = Divide(x=w61, y=w60) -> (x/y=w219:dbl)
  n163 = Divide(x=w61, y=w60) -> (x/y=w234:dbl)
  n164 = Subtract(x=w62, y=w52) -> (x-y=w267:dbl)
  n165 = Subtract(x=w62, y=w53) -> (x-y=w251:dbl)
  n166 = Divide(x=w61, y=w60) -> (x/y=w266:dbl)
  n167 = Divide(x=w61, y=w60) -> (x/y=w250:dbl)
  n168 = Multiply(x=w220, y=w219) -> (x*y=→"Rotation steering angle 4":dbl)
  n169 = Multiply(x=w235, y=w234) -> (x*y=→"Rotation steering angle 3":dbl)
  n170 = Negate(x=w34) -> (-x=w174:dbl)
  n171 = Multiply(x=w267, y=w266) -> (x*y=→"Rotation steering angle 1":dbl)
  n172 = Multiply(x=w251, y=w250) -> (x*y=→"Rotation steering angle 2":dbl)
  n173 = Cosine(x=w220) -> (cos(x)=w218:dbl)
  n174 = Sine(x=w220) -> (sin(x)=w217:dbl)
  n175 = Negate(x=w34) -> (-x=w175:dbl)
  n176 = Cosine(x=w235) -> (cos(x)=w233:dbl)
  n177 = Sine(x=w235) -> (sin(x)=w232:dbl)
  n178 = Cosine(x=w267) -> (cos(x)=w264:dbl)
  n179 = Cosine(x=w251) -> (cos(x)=w248:dbl)
  n180 = Sine(x=w267) -> (sin(x)=w263:dbl)
  n181 = Sine(x=w251) -> (sin(x)=w247:dbl)
  n182 = Multiply(x=w34, y=w217) -> (x*y=w216:dbl)
  n183 = Multiply(x=w34, y=w218) -> (x*y=w215:dbl)
  n184 = Multiply(x=w34, y=w232) -> (x*y=w231:dbl)
  n185 = Multiply(x=w34, y=w233) -> (x*y=w230:dbl)
  n186 = Multiply(x=w175, y=w263) -> (x*y=w262:dbl)
  n187 = Multiply(x=w175, y=w264) -> (x*y=w261:dbl)
  n188 = Multiply(x=w174, y=w247) -> (x*y=w246:dbl)
  n189 = Multiply(x=w174, y=w248) -> (x*y=w245:dbl)
  n190 = Add(x=w211, y=w216) -> (x+y=w214:dbl)
  "X4" <- w214
  n191 = Add(x=w212, y=w215) -> (x+y=w213:dbl)
  "Y4" <- w213
  n192 = Add(x=w211, y=w231) -> (x+y=w229:dbl)
  "X3" <- w229
  n193 = Add(x=w212, y=w230) -> (x+y=w228:dbl)
  "Y3" <- w228
  n194 = Add(x=w211, y=w262) -> (x+y=w260:dbl)
  "X1" <- w260
  n195 = Add(x=w212, y=w261) -> (x+y=w259:dbl)
  "Y1" <- w259
  n196 = Add(x=w211, y=w246) -> (x+y=w244:dbl)
  "X2" <- w244
  n197 = Add(x=w212, y=w245) -> (x+y=w243:dbl)
  "Y2" <- w243
  n198 = Square(x=w214) -> (x^2=w227:dbl)
  n199 = Square(x=w213) -> (x^2=w225:dbl)
  n200 = Square(x=w229) -> (x^2=w242:dbl)
  n201 = Square(x=w228) -> (x^2=w240:dbl)
  n202 = Inverse Tangent (2 Input)(1:w213, 2:w214) -> (0:w223:dbl)
  n203 = Inverse Tangent (2 Input)(1:w228, 2:w229) -> (0:w238:dbl)
  n204 = Square(x=w260) -> (x^2=w274:dbl)
  n205 = Square(x=w259) -> (x^2=w272:dbl)
  n206 = Square(x=w244) -> (x^2=w258:dbl)
  n207 = Square(x=w243) -> (x^2=w256:dbl)
  n208 = Inverse Tangent (2 Input)(1:w259, 2:w260) -> (0:w270:dbl)
  n209 = Inverse Tangent (2 Input)(1:w243, 2:w244) -> (0:w254:dbl)
  n210 = Add(x=w227, y=w225) -> (x+y=w226:dbl)
  n211 = Add(x=w242, y=w240) -> (x+y=w241:dbl)
  n212 = Add(x=w274, y=w272) -> (x+y=w273:dbl)
  n213 = Add(x=w258, y=w256) -> (x+y=w257:dbl)
  n214 = Divide(x=180.0, y=3.141592653589793) -> (x/y=w224:dbl)
  n215 = Divide(x=180.0, y=3.141592653589793) -> (x/y=w239:dbl)
  n216 = Divide(x=180.0, y=3.141592653589793) -> (x/y=w271:dbl)
  n217 = Divide(x=180.0, y=3.141592653589793) -> (x/y=w255:dbl)
  n218 = Square Root(x=w226) -> (sqrt(x)=w127:dbl)
  n219 = Multiply(x=w224, y=w223) -> (x*y=w128:dbl)
  n220 = Square Root(x=w241) -> (sqrt(x)=w139:dbl)
  n221 = Multiply(x=w239, y=w238) -> (x*y=w141:dbl)
  n222 = Square Root(x=w273) -> (sqrt(x)=w164:dbl)
  n223 = Multiply(x=w271, y=w270) -> (x*y=w169:dbl)
  n224 = Square Root(x=w257) -> (sqrt(x)=w152:dbl)
  n225 = Multiply(x=w255, y=w254) -> (x*y=w155:dbl)
  n226 = Divide(x=360.0 ("y"), y=w159) -> (x/y=w158:dbl)
  n227 = Divide(x=360.0 ("y"), y=w170) -> (x/y=w104:dbl)
  n228 = Divide(x=360.0 ("y"), y=w145) -> (x/y=w144:dbl)
  n229 = Divide(x=360.0 ("y"), y=w132) -> (x/y=w131:dbl)
  n230 = Divide(x=w181, y=360.0) -> (x/y=w182:dbl)
  n231 = Divide(x=w105, y=360.0) -> (x/y=w193:dbl)
  n232 = Divide(x=w185, y=360.0) -> (x/y=w186:dbl)
  n233 = Divide(x=w189, y=360.0) -> (x/y=w190:dbl)
  n234 = call <vilib>:"CTRE_Phoenix_MotorControl_RefNumRegistryGet.vi"("refnum name"="Blue Front Drive") -> ("error out"=w111:errorcluster, "PhoenixMotorControlDevRef"=w206:T6)  [unwired: 9 in]
  n235 = call <vilib>:"CTRE_Phoenix_MotorControl_RefNumRegistryGet.vi"("refnum name"="Orange Front Drive") -> ("error out"=w110:errorcluster, "PhoenixMotorControlDevRef"=w203:T6)  [unwired: 9 in]
  n236 = call <vilib>:"CTRE_Phoenix_MotorControl_RefNumRegistryGet.vi"("refnum name"="Orange Back Drive") -> ("error out"=w113:errorcluster, "PhoenixMotorControlDevRef"=w210:T6)  [unwired: 9 in]
  n237 = call <vilib>:"CTRE_Phoenix_MotorControl_RefNumRegistryGet.vi"("refnum name"="Blue Back Drive") -> ("error out"=w112:errorcluster, "PhoenixMotorControlDevRef"=w207:T6)  [unwired: 9 in]
  n238 = call <vilib>:"CTRE_Phoenix_MotorControl_RefNumRegistryGet.vi"("refnum name"="Orange Back Turn") -> ("error out"=w109:errorcluster, "PhoenixMotorControlDevRef"=w201:T6)  [unwired: 9 in]
  n239 = call <vilib>:"CTRE_Phoenix_MotorControl_RefNumRegistryGet.vi"("refnum name"="Orange Front Turn") -> ("error out"=w106:errorcluster, "PhoenixMotorControlDevRef"=w198:T6)  [unwired: 9 in]
  n240 = call <vilib>:"CTRE_Phoenix_MotorControl_RefNumRegistryGet.vi"("refnum name"="Blue Back Turn") -> ("error out"=w108:errorcluster, "PhoenixMotorControlDevRef"=w200:T6)  [unwired: 9 in]
  n241 = call <vilib>:"CTRE_Phoenix_MotorControl_RefNumRegistryGet.vi"("refnum name"="Blue Front Turn") -> ("error out"=w107:errorcluster, "PhoenixMotorControlDevRef"=w199:T6)  [unwired: 9 in]
  n242 = call <vilib>:"CTRE_Phoenix_CANcoder_RefNumRegistryGet.vi"("refnum name"="Blue Front Cancoder") -> ("error out"=w94:errorcluster, "CTRE_CANcoder_DeviceRef"=w95:T23)  [unwired: 9 in]
  n243 = call <vilib>:"CTRE_Phoenix_CANcoder_RefNumRegistryGet.vi"("refnum name"="Orange Back Cancoder") -> ("error out"=w100:errorcluster, "CTRE_CANcoder_DeviceRef"=w101:T23)  [unwired: 9 in]
  n244 = call <vilib>:"CTRE_Phoenix_CANcoder_RefNumRegistryGet.vi"("refnum name"="Orange Front Cancoder") -> ("error out"=w91:errorcluster, "CTRE_CANcoder_DeviceRef"=w92:T23)  [unwired: 9 in]
  n245 = call <vilib>:"CTRE_Phoenix_CANcoder_RefNumRegistryGet.vi"("refnum name"="Blue Back Cancoder") -> ("error out"=w97:errorcluster, "CTRE_CANcoder_DeviceRef"=w98:T23)  [unwired: 9 in]
  n246 = call-poly <vilib>:"CTRE_Phoenix_CANcoder_GetPolymorphic.vi"("CTRE_CANcoder_DeviceRef"=w95, "error in"=w94) -> ("Position"=w64:dbl)  [unwired: 9 in, 4 out]
  n247 = call-poly <vilib>:"CTRE_Phoenix_CANcoder_GetPolymorphic.vi"("CTRE_CANcoder_DeviceRef"=w101, "error in"=w100) -> ("Position"=w49:dbl)  [unwired: 9 in, 4 out]
  n248 = call-poly <vilib>:"CTRE_Phoenix_CANcoder_GetPolymorphic.vi"("CTRE_CANcoder_DeviceRef"=w92, "error in"=w91) -> ("Position"=w63:dbl)  [unwired: 9 in, 4 out]
  n249 = call-poly <vilib>:"CTRE_Phoenix_CANcoder_GetPolymorphic.vi"("CTRE_CANcoder_DeviceRef"=w98, "error in"=w97) -> ("Position"=w65:dbl)  [unwired: 9 in, 4 out]
  n250 = feedback #7() -> (w48:dbl)  [unwired: 1 in]
  "Sensor Position 2" <- w48
  n251 = feedback-in #7(w65) -> ()
  n252 = feedback #8() -> (w30:dbl)  [unwired: 1 in]
  "Sensor Position 1" <- w30
  n253 = feedback-in #8(w49) -> ()
  n254 = feedback #9() -> (w46:dbl)  [unwired: 1 in]
  "Sensor Position 3" <- w46
  n255 = feedback-in #9(w64) -> ()
  n256 = Add(x=w30, y=0.0) -> (x+y=w28:dbl)
  n257 = Multiply(x=w104, y=w28) -> (x*y=w55:dbl)
  n258 = Divide(x=w55, y=12.8 ("x")) -> (x/y=w84:dbl)
  n259 = Add(x=180.0, y=w84) -> (x+y=w173:dbl)
  n260 = call "Angle Distance VI.vi"("current angle"=w173, "target angle"=w169) -> ("distance"=w165:dbl)  [unwired: 9 in]
  n261 = call "Angle Distance VI.vi"("current angle"=w84, "target angle"=w169) -> ("distance"=w166:dbl)  [unwired: 9 in]
  n262 = Absolute Value(x=w166) -> (abs(x)=w168:dbl)
  n263 = Greater?(x=w168, y=90.0 ("x")) -> (0:w89:bool)
  n264 = case shown="True" w89 {
    tunnel: w166 -> [w565 _]
    tunnel: [w565 w568] -> w103
    tunnel: w165 -> [_ w568]
    tunnel: w164 -> [w564 w567]
    tunnel: [w564 w566] -> w163
    frame False {
    }
    frame True {
      n265 = Negate(x=w567) -> (-x=w566:dbl)
    }
  }
  "WheelDirection1" <- w103
  n266 = Multiply(x=w103, y=w193) -> (x*y=w86:dbl)
  n267 = Divide(x=w86, y=12.8) -> (x/y=w27:dbl)
  "Desired Position 1" <- w27
  n268 = call-poly <vilib>:"PID.vi"("output range"=cluster{"output high":dbl, "output low":dbl} {"output high"=0.5, "output low"=-0.5}, "PID gains"="PID gains", "process variable"=w28, "setpoint"=w27) -> ("output"=w29:dbl)  [unwired: 6 in, 1 out]
  "Motor out 1" <- w29
  n269 = call <vilib>:"CTRE_Phoenix_MotorControl_Set.vi"("error in (no error)"=w109, "Output"=w29, "Control Mode"=w102, "PhoenixMotorControlDevRef"=w201) -> ()  [unwired: 6 in, 2 out]
  n270 = feedback #10() -> (w43:dbl)  [unwired: 1 in]
  "Sensor Position 4" <- w43
  n271 = feedback-in #10(w63) -> ()
  n272 = Add(x=w48, y=0.0) -> (x+y=w32:dbl)
  n273 = Multiply(x=w158, y=w32) -> (x*y=w73:dbl)
  n274 = Divide(x=w73, y=12.8) -> (x/y=w72:dbl)
  n275 = Add(x=180.0, y=w72) -> (x+y=w162:dbl)
  n276 = call "Angle Distance VI.vi"("current angle"=w162, "target angle"=w155) -> ("distance"=w153:dbl)  [unwired: 9 in]
  n277 = call "Angle Distance VI.vi"("current angle"=w72, "target angle"=w155) -> ("distance"=w150:dbl)  [unwired: 9 in]
  n278 = Absolute Value(x=w150) -> (abs(x)=w157:dbl)
  n279 = Greater?(x=w157, y=90.0 ("x")) -> (0:w154:bool)
  n280 = case shown="True" w154 {
    tunnel: w150 -> [w570 _]
    tunnel: [w570 w573] -> w149
    tunnel: w153 -> [_ w573]
    tunnel: w152 -> [w569 w572]
    tunnel: [w569 w571] -> w151
    frame False {
    }
    frame True {
      n281 = Negate(x=w572) -> (-x=w571:dbl)
    }
  }
  "WheelDirection2" <- w149
  n282 = Multiply(x=w149, y=w190) -> (x*y=w82:dbl)
  n283 = Divide(x=w82, y=12.8) -> (x/y=w81:dbl)
  "Desired Position 2" <- w81
  n284 = call-poly <vilib>:"PID.vi"("output range"=cluster{"output high":dbl, "output low":dbl} {"output high"=0.5, "output low"=-0.5}, "PID gains"="PID gains 2", "process variable"=w32, "setpoint"=w81) -> ("output"=w177:dbl)  [unwired: 6 in, 1 out]
  "Motor Out 2" <- w177
  n285 = call <vilib>:"CTRE_Phoenix_MotorControl_Set.vi"("error in (no error)"=w108, "Output"=w177, "Control Mode"=w116, "PhoenixMotorControlDevRef"=w200) -> ()  [unwired: 6 in, 2 out]
  n286 = Add(x=w46, y=0.0) -> (x+y=w31:dbl)
  n287 = Multiply(x=w144, y=w31) -> (x*y=w70:dbl)
  n288 = Divide(x=w70, y=12.8) -> (x/y=w69:dbl)
  n289 = Add(x=180.0, y=w69) -> (x+y=w148:dbl)
  n290 = call "Angle Distance VI.vi"("current angle"=w148, "target angle"=w141) -> ("distance"=w140:dbl)  [unwired: 9 in]
  n291 = call "Angle Distance VI.vi"("current angle"=w69, "target angle"=w141) -> ("distance"=w137:dbl)  [unwired: 9 in]
  n292 = Absolute Value(x=w137) -> (abs(x)=w143:dbl)
  n293 = Greater?(x=w143, y=90.0 ("x")) -> (0:w121:bool)
  n294 = case shown="True" w121 {
    tunnel: w137 -> [w575 _]
    tunnel: [w575 w578] -> w136
    tunnel: w140 -> [_ w578]
    tunnel: w139 -> [w574 w577]
    tunnel: [w574 w576] -> w138
    frame False {
    }
    frame True {
      n295 = Negate(x=w577) -> (-x=w576:dbl)
    }
  }
  "WheelDirection3" <- w136
  n296 = Multiply(x=w136, y=w186) -> (x*y=w78:dbl)
  n297 = Divide(x=w78, y=12.8) -> (x/y=w79:dbl)
  "Desired Position 3" <- w79
  n298 = call-poly <vilib>:"PID.vi"("output range"=cluster{"output high":dbl, "output low":dbl} {"output high"=0.5, "output low"=-0.5}, "PID gains"="PID gains 3", "process variable"=w31, "setpoint"=w79) -> ("output"=w178:dbl)  [unwired: 6 in, 1 out]
  "Motor out 3" <- w178
  n299 = call <vilib>:"CTRE_Phoenix_MotorControl_Set.vi"("error in (no error)"=w107, "Output"=w178, "Control Mode"=w117, "PhoenixMotorControlDevRef"=w199) -> ()  [unwired: 6 in, 2 out]
  n300 = Add(x=w43, y=0.0) -> (x+y=w42:dbl)
  n301 = Multiply(x=w131, y=w42) -> (x*y=w67:dbl)
  n302 = Divide(x=w67, y=12.8) -> (x/y=w66:dbl)
  n303 = Add(x=180.0, y=w66) -> (x+y=w135:dbl)
  n304 = call "Angle Distance VI.vi"("current angle"=w135, "target angle"=w128) -> ("distance"=w124:dbl)  [unwired: 9 in]
  n305 = call "Angle Distance VI.vi"("current angle"=w66, "target angle"=w128) -> ("distance"=w123:dbl)  [unwired: 9 in]
  n306 = Absolute Value(x=w123) -> (abs(x)=w130:dbl)
  n307 = Greater?(x=w130, y=90.0 ("x")) -> (0:w125:bool)
  n308 = case shown="True" w125 {
    tunnel: w123 -> [w580 _]
    tunnel: [w580 w583] -> w122
    tunnel: w124 -> [_ w583]
    tunnel: w127 -> [w579 w582]
    tunnel: [w579 w581] -> w126
    frame False {
    }
    frame True {
      n309 = Negate(x=w582) -> (-x=w581:dbl)
    }
  }
  "WheelDirection4" <- w122
  n310 = call <vilib>:"WPI_RobotDriveNormalize 4.vi"("D"=w126, "C"=w138, "B"=w151, "A"=w163) -> ("D'"=w33:dbl, "C'"=w202:dbl, "B'"=w37:dbl, "A'"=w26:dbl)
  "Throttle 1" <- w26
  "Throttle 2" <- w37
  "Throttle 3" <- w202
  "Throttle 4" <- w33
  "frontleftdrive" <- w33
  "frontrightmotor" <- w202
  n311 = Multiply(x=w122, y=w182) -> (x*y=w75:dbl)
  n312 = Divide(x=w75, y=12.8) -> (x/y=w76:dbl)
  "Desired Position 4" <- w76
  n313 = call <vilib>:"CTRE_Phoenix_MotorControl_Set.vi"("error in (no error)"=w111, "Output"=w202, "Control Mode"=w120, "PhoenixMotorControlDevRef"=w206) -> ()  [unwired: 6 in, 2 out]
  n314 = call <vilib>:"CTRE_Phoenix_MotorControl_Set.vi"("error in (no error)"=w113, "Output"=w26, "Control Mode"=w114, "PhoenixMotorControlDevRef"=w210) -> ()  [unwired: 6 in, 2 out]
  n315 = call <vilib>:"CTRE_Phoenix_MotorControl_Set.vi"("error in (no error)"=w110, "Output"=w33, "Control Mode"=w119, "PhoenixMotorControlDevRef"=w203) -> ()  [unwired: 6 in, 2 out]
  n316 = call <vilib>:"CTRE_Phoenix_MotorControl_Set.vi"("error in (no error)"=w112, "Output"=w37, "Control Mode"=w115, "PhoenixMotorControlDevRef"=w207) -> ()  [unwired: 6 in, 2 out]
  n317 = call-poly <vilib>:"PID.vi"("output range"=cluster{"output high":dbl, "output low":dbl} {"output high"=0.5, "output low"=-0.5}, "PID gains"="PID gains 4", "process variable"=w42, "setpoint"=w76) -> ("output"=w176:dbl)  [unwired: 6 in, 1 out]
  "Motor out 4" <- w176
  n318 = call <vilib>:"CTRE_Phoenix_MotorControl_Set.vi"("error in (no error)"=w106, "Output"=w176, "Control Mode"=w118, "PhoenixMotorControlDevRef"=w198) -> ()  [unwired: 6 in, 2 out]
